vi "Start Point.vi"(7 "Point Ident":string, 8 "error in":errorcluster, 11 "MSS Target Actor in":refnum<class "MSS Target Actor.lvclass">) -> (0 "error out":errorcluster, 3 "MSS Target Actor out":refnum<class "MSS Target Actor.lvclass">)   [LabVIEW 2023, in "MSS Target Actor.lvlib" / "MSS Target Actor.lvclass"]
uses:
  MSS Target Actor.lvclass
  MSS Target Actor.lvclass/MSS Target Actor.ctl
  Measure and Stimulus Subsystems/Measure and Stimulus Subsystems.lvclass
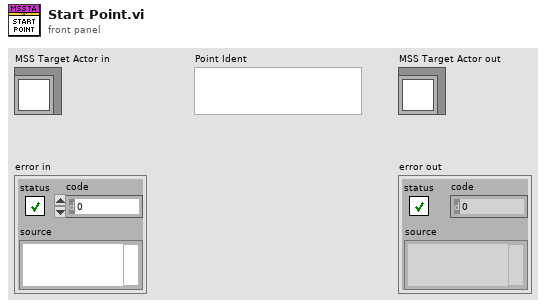
[diagram p1: front panel]
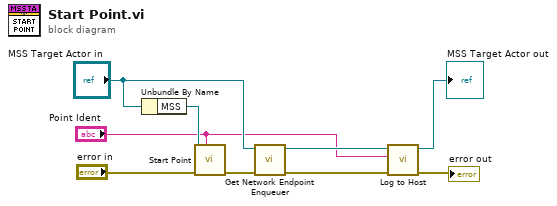
[diagram p0: block diagram]
diagram:
  n1 = Unbundle By Name("MSS Target Actor in") -> ("MSS"=w9:refnum<class "Measure and Stimulus Subsystems.lvclass">)
  n2 = call "Start Point.vi"("Point Ident"="Point Ident", "error in"="error in", "MSS in"=w9) -> ("error out"=w7:errorcluster)  [unwired: 7 in, 1 out]
  n3 = call "Get Network Endpoint Enqueuer.vi"("error in"=w7, "MSS Target Actor in"="MSS Target Actor in") -> ("error out"=w5:errorcluster, "MSS Target Actor out"=w3:refnum<class "MSS Target Actor.lvclass">)  [unwired: 6 in, 2 out]
  n4 = call "Log to Host.vi"("error in"=w5, "Detail"="Point Ident", "MSS Target Actor in"=w3) -> ("error out"=→"error out":errorcluster, "MSS Target Actor out"=→"MSS Target Actor out":refnum<class "MSS Target Actor.lvclass">)  [unwired: 7 in]
